vi "Configure Arbitrary Waveform Trigger Source.vi"(8 "error in (no error)":errorcluster, 10 "Acquisition Trigger Source (0: Bus)":u16(ring) items=["Bus", "External", "Immediate", "Pin 1", "Pin 2", "Pin 3", "Pin 4", "Pin 5", "Pin 6", "Pin 7"], 11 "VISA resource name":refnum<visa-resource-name>) -> (0 "error out":errorcluster, 3 "VISA resource name out":refnum<visa-resource-name>)   [LabVIEW 2021, in "Agilent N6900 N7900 Series.lvlib"]
doc: "Selects the trigger source for arbitrary waveforms."
uses:
  <instrlib>/Agilent N6900 N7900 Series/Agilent N6900 N7900 Series.lvlib
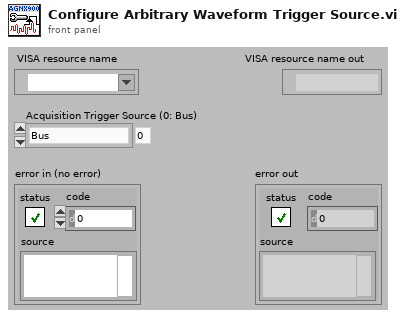
[diagram p1: front panel]
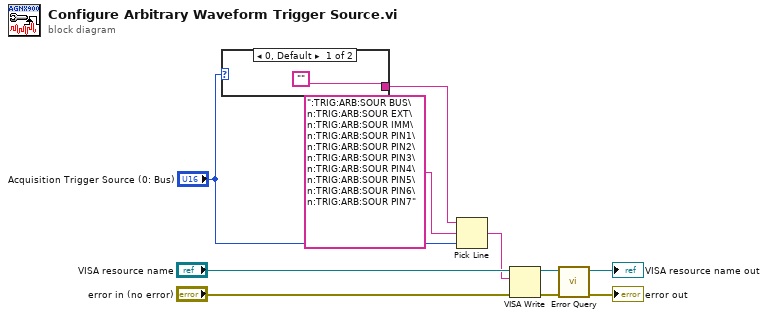
[diagram p0: block diagram]
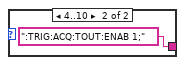
[diagram p2: hidden frame]
diagram:
  n1 = case shown="0, Default" "Acquisition Trigger Source (0: Bus)" {
    tunnel: ["" ("string (\"\")") ":TRIG:ACQ:TOUT:ENAB 1;" ("string (\"\")")] -> w1
    frame 0, Default {
    }
    frame 4..10 {
    }
  }
  n2 = Pick Line(string ("")=w1, multi-line string=":TRIG:ARB:SOUR BUS\n:TRIG:ARB:SOUR EXT\n:TRIG:ARB:SOUR IMM\n:TRIG:ARB:SOUR PIN1\n:TRIG:ARB:SOUR PIN2\n:TRIG:ARB:SOUR PIN3\n:TRIG:ARB:SOUR PIN4\n:TRIG:ARB:SOUR PIN5\n:TRIG:ARB:SOUR PIN6\n:TRIG:ARB:SOUR PIN7", line index="Acquisition Trigger Source (0: Bus)") -> (output string=w4:string)
  n3 = VISA Write(VISA resource name="VISA resource name", write buffer=w4, error in (no error)="error in (no error)") -> (VISA resource name out=w7:refnum<visa-resource-name>, error out=w8:errorcluster)  [unwired: 1 out]
  n4 = call <instrlib>:"Error Query.vi"("error in (no error)"=w8, "VISA resource name"=w7) -> ("error out"=→"error out":errorcluster, "VISA resource name out"=→"VISA resource name out":refnum<visa-resource-name>)  [unwired: 6 in, 2 out]
